vi "CH_LM App DataFileHeader.vi"(1 "Data format":u16, 2 "Meter Info":cluster{"Probe Type":T1, "Probe Qualifier":T2}[](array[cluster]), 3 "Serial Numbers":string) -> (0 "Header":string)   [LabVIEW 2012, in "CH_LM App.lvlib"]
doc: "This VI constructs the Data File Header."
uses:
  CH_LM App.lvlib
  CH_LM.lvlib
  CH_LM/CH_LM ProbeType.ctl
  CH_LM/CH_LM ProbeQualifier.ctl
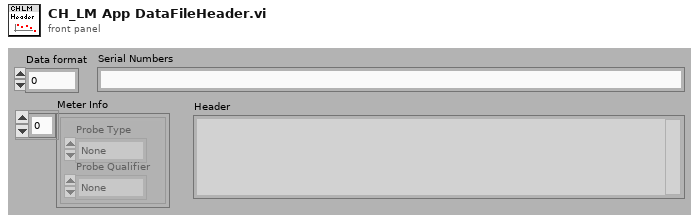
[diagram p1: front panel]
types:
  T1 = typedef "CH_LM.lvlib/CH_LM ProbeType.ctl" = enum16{"None", "Thermopile", "Pyroelectric", "Optical"}
  T2 = typedef "CH_LM.lvlib/CH_LM ProbeQualifier.ctl" = enum16{"None", "Single", "Quad", "No Spec"}
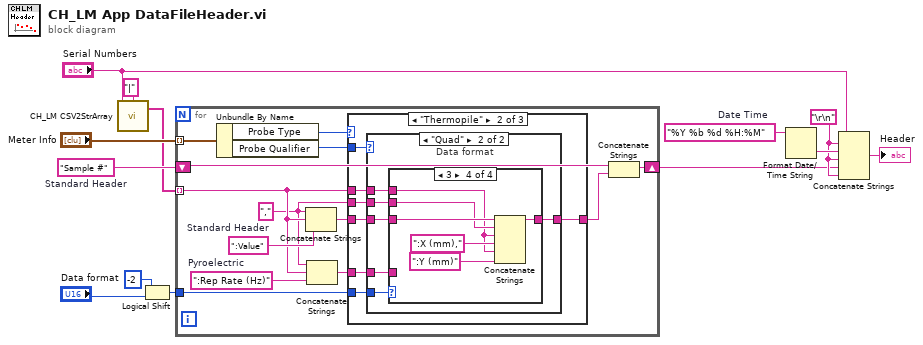
[diagram p0: block diagram]
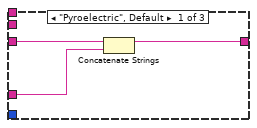
[diagram p2: hidden frame]
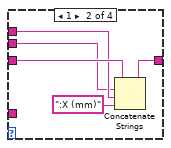
[diagram p5: hidden frame]
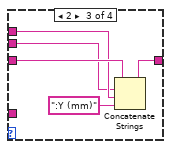
[diagram p6: hidden frame]
diagram:
  w4 = "Sample #"  # Standard Header
  w12 = "%Y %b %d %H:%M"  # Date Time
  w10 = "\r\n" ("End of Line Constant")
  n1 = call "CH_LM CSV2StrArray.vi"("CSL"="Serial Numbers", "Separator (,)"="|") -> ("Strings"=w1:string[])  [unwired: 1 in, 1 out]
  n2 = Logical Shift(y=i16 -2, x="Data format") -> (x << y=w6:u16)
  n3 = for {
    tunnel: "Meter Info" -> [w23] mode=indexing
    shift-right: [w25] -> w5
    shift-left: w4 -> [w26]
    tunnel: w6 -> [w20]
    tunnel: w1 -> [w15] mode=indexing
    w14 = "," ("string")
    w17 = ":Rep Rate (Hz)"  # Pyroelectric
    w19 = ":Value"  # Standard Header
    n4 = Unbundle By Name(w23) -> ("Probe Type"=w22:T1, "Probe Qualifier"=w21:T2)
    n5 = Concatenate Strings(w14, w15, w19) -> (w18:string)
    n6 = Concatenate Strings(w14, w15, w17) -> (w16:string)
    n7 = case shown="\"Thermopile\"" w22 {
      tunnel: [w27 w35 w61] -> w24
      tunnel: w18 -> [w29 w36 w61]
      tunnel: w21 -> [_ w33 _]
      tunnel: w16 -> [w28 w34 _]
      tunnel: w20 -> [_ w32 _]
      tunnel: w15 -> [_ w31 _]
      tunnel: w14 -> [_ w30 _]
      frame "Pyroelectric", Default {
        n8 = Concatenate Strings(w29, w28) -> (w27:string)
      }
      frame "Thermopile" {
        n9 = case shown="\"Quad\"" w33 {
          tunnel: w36 -> [w37 w43]
          tunnel: [w37 w42] -> w35
          tunnel: w34 -> [_ w41]
          tunnel: w32 -> [_ w40]
          tunnel: w31 -> [_ w39]
          tunnel: w30 -> [_ w38]
          frame "Single", Default {
          }
          frame "Quad" {
            n10 = case "Data format" shown="3" w40 {
              tunnel: w43 -> [w44 w49 w54 w60]
              tunnel: [w44 w48 w53 w59] -> w42
              tunnel: w41 -> [_ _ _ _]
              tunnel: w39 -> [_ w46 w51 w56]
              tunnel: w38 -> [_ w45 w50 w57]
              frame 0, Default {
              }
              frame 1 {
                n11 = Concatenate Strings(w49, w45, w46, ":X (mm)" ("string")) -> (w48:string)
              }
              frame 2 {
                n12 = Concatenate Strings(w54, w50, w51, ":Y (mm)" ("string")) -> (w53:string)
              }
              frame 3 {
                n13 = Concatenate Strings(w60, w57, w56, ":X (mm)," ("string"), w56, ":Y (mm)" ("string")) -> (w59:string)
              }
            }
          }
        }
      }
      frame "Optical" {
      }
    }
    n14 = Concatenate Strings(w26, w24) -> (w25:string)
  }
  n15 = Format Date/Time String(time format string (%c)=w12) -> (date/time string=w11:string)  [unwired: 2 out]
  n16 = Concatenate Strings("Serial Numbers", w10, w11, w10, w5, w10) -> (→"Header":string)
